vi "Create Level.vi"(8 "Error In":errorcluster, 10 "Selected Level":string, 11 "WAD Cluster IN":T1) -> (0 "Error Out":errorcluster, 2 "2D Picture":picture, 3 "WAD Cluster OUT":T1)   [LabVIEW 2017]
uses:
  WAD_MainCluster.ctl
  TextureList.ctl
  PatchList.ctl
  Lumps.ctl
  THINGSList.ctl
  <userlib>/_OpenG.lib/array/array.llb/Search 1D Array (String)__ogtk.vi
  <userlib>/_OpenG.lib/array/array.llb/Delete Elements from 1D Array (String)__ogtk.vi
  <userlib>/_OpenG.lib/array/array.llb/Filter 1D Array with Scalar (I32)__ogtk.vi
  <vilib>/picture/picture.llb/Draw 8-Bit Pixmap.vi
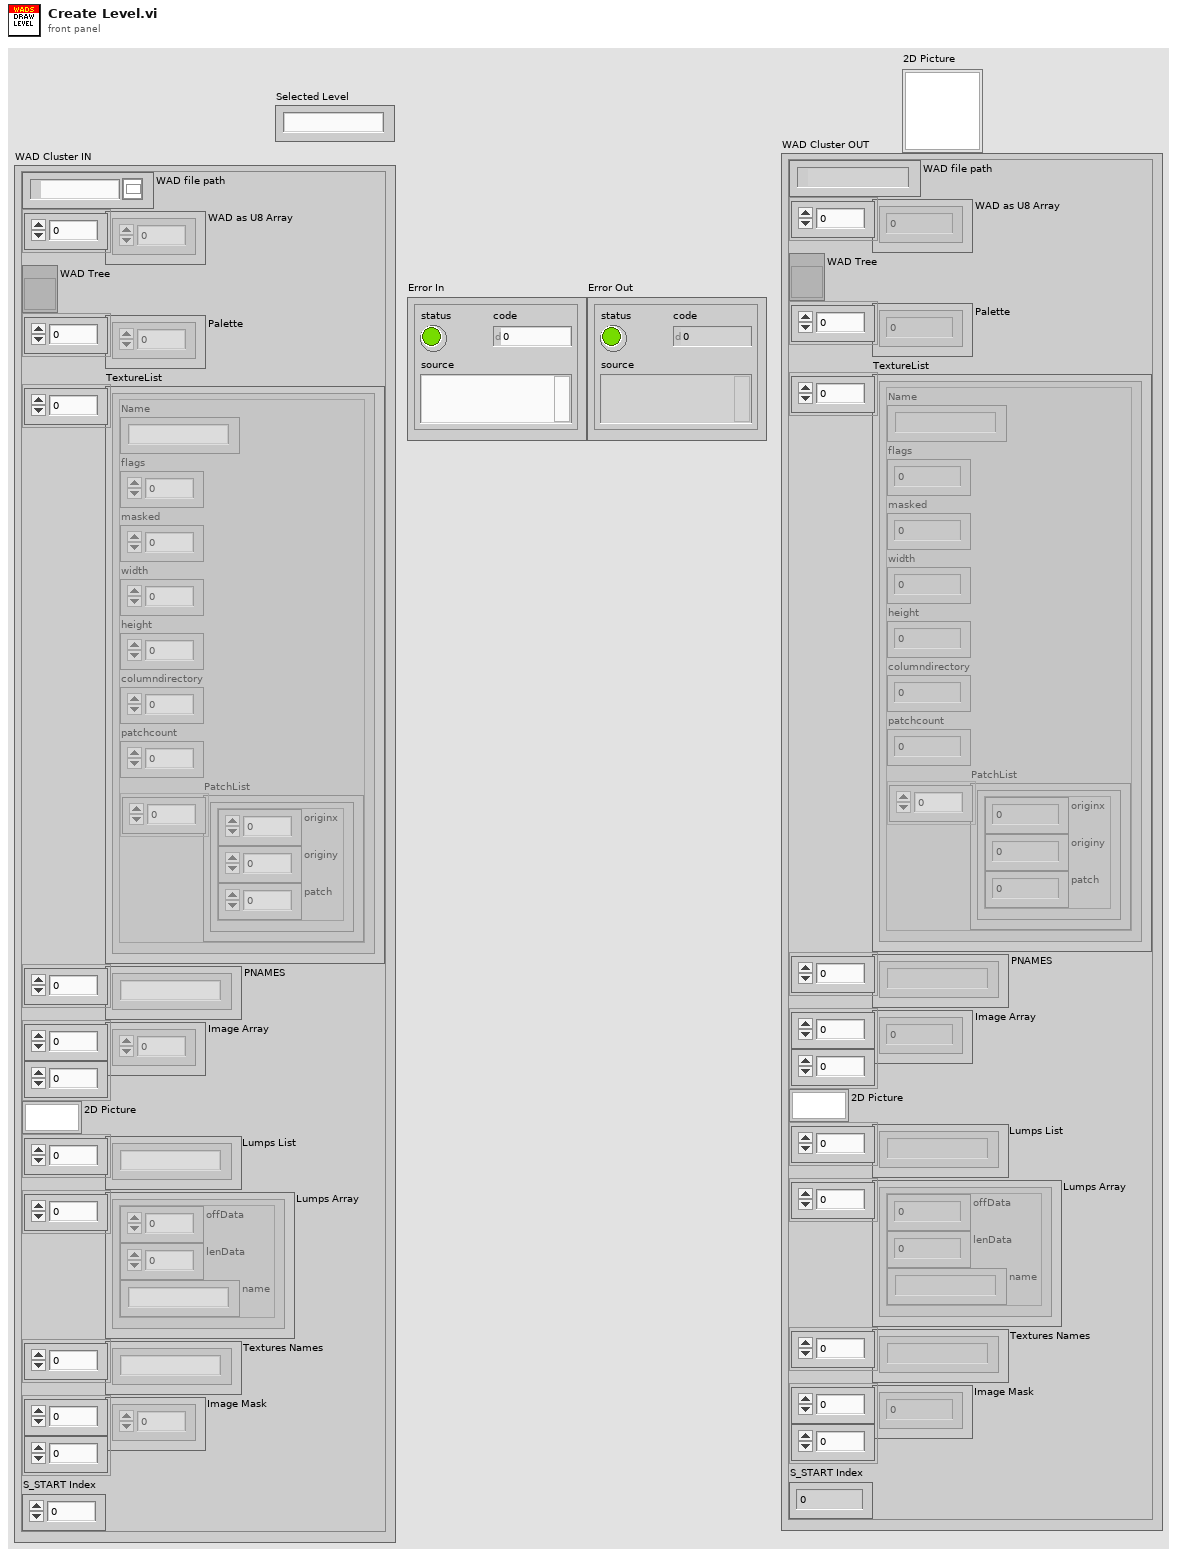
[diagram p1: front panel]
types:
  T1 = typedef "WAD_MainCluster.ctl" = cluster{"WAD file path":path, "WAD as U8 Array":u8[], "WAD Tree":refnum<vi>, "Palette":u32[], "TextureList":T2[], "PNAMES":string[], "Image Array":i16[][], "2D Picture":picture, "Lumps List":string[], "Lumps Array":T4[], "Textures Names":string[], "Image Mask":i16[][], "S_START Index":i32}
  T2 = typedef "TextureList.ctl" = cluster{"Name":string, "flags":u16, "masked":i16, "width":i16, "height":i16, "columndirectory":u32, "patchcount":i16, "PatchList":T3[]}
  T3 = typedef "PatchList.ctl" = cluster{"originx":i16, "originy":i16, "patch":i16}
  T4 = typedef "Lumps.ctl" = cluster{"offData":i32, "lenData":i32, "name":string}
  T5 = cluster{"left":i16, "top":i16, "right":i16, "bottom":i16}
  T6 = typedef "THINGSList.ctl" = string[][]
  T7 = cluster{"filtered array[0]":i32, "filtered array[1]":i32}
  T8 = typedef "PatchHeader.ctl" = cluster{"Width":u16, "Height":u16, "XOffset":i16, "YOffset":i16}
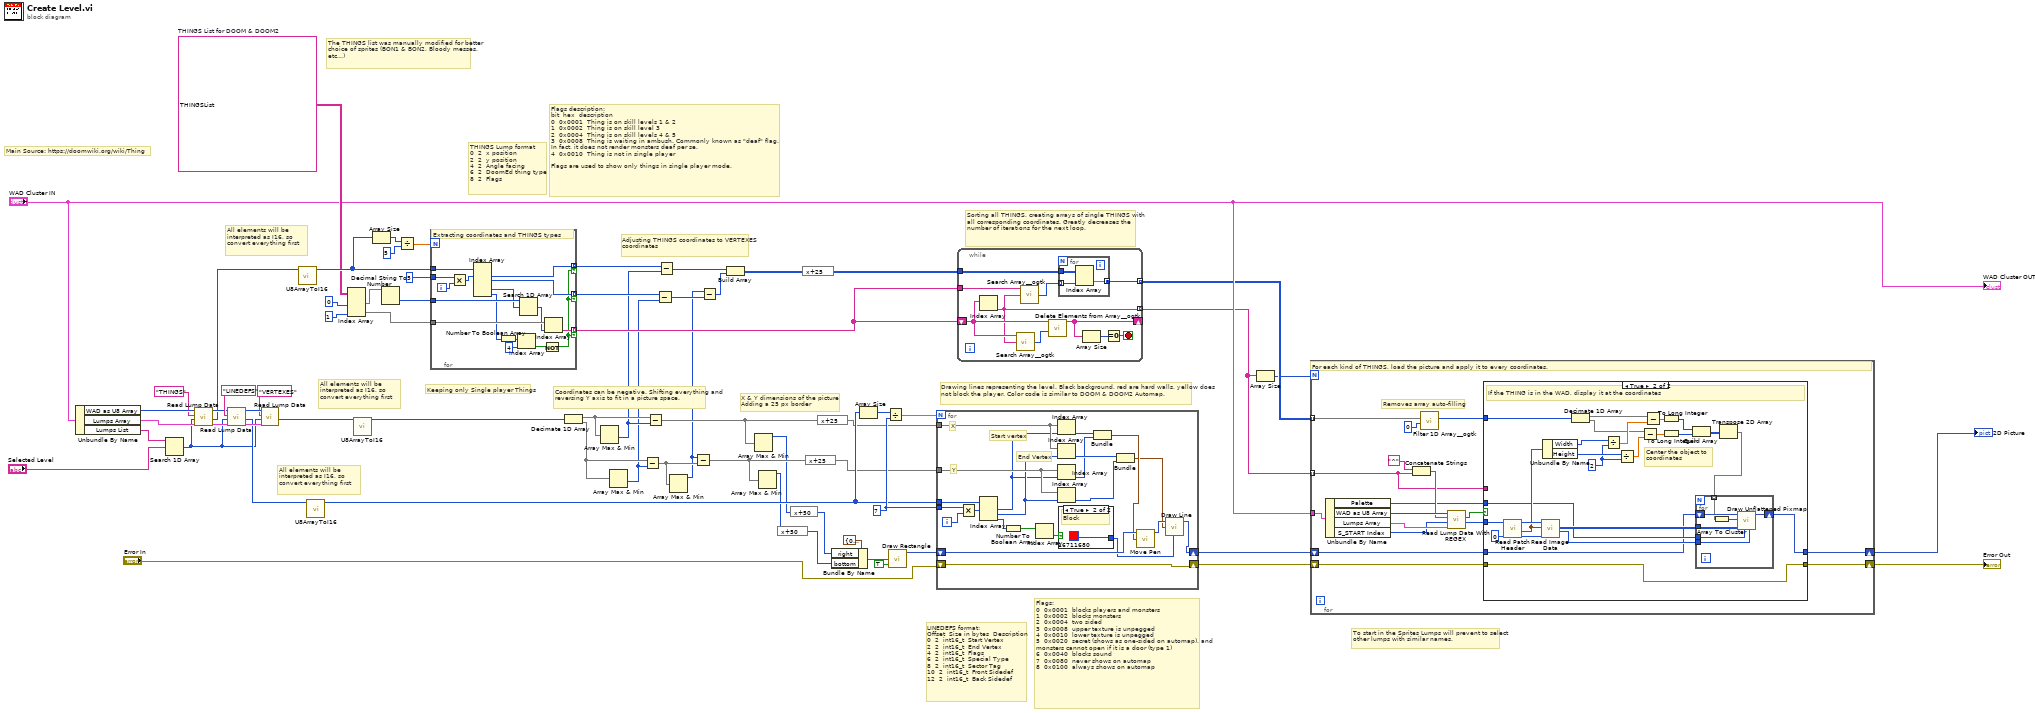
[diagram p0: block diagram]
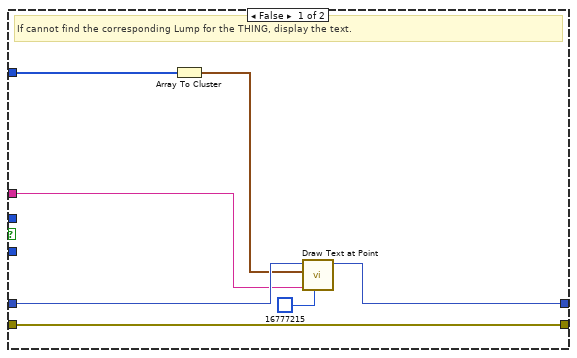
[diagram p2: hidden frame]
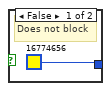
[diagram p3: hidden frame]
diagram:
  w21 = T6 [["1", "PLAY"], ["2", "PLAY"], ["3", "PLAY"], ["4", "PLAY"], ["5", "BKEY"], ["6", "YKEY"], ["7", "SPID"], ["8", "BPAK"], ["9", "SPOS"], ["10", "PLAYN"], ["11", "DM Spawn"], ["12", "PLAYW"], ["13", "RKEY"], ["14", "Teleport"], ["15", "PLAYN"], ["16", "CYBR"], ["17", "CELP"], ["18", "POSSL"], ["19", "SPOSL"], ["20", "TROOM"], ["21", "SARGN"], ["22", "HEADL"], ["23", "SKUL"], ["24", "POL5"], ["25", "POL1"], ["26", "POL6"], ["27", "POL4"], ["28", "POL2"], ["29", "POL3"], ["30", "COL1"], ["31", "COL2"], ["32", "COL3"], ["33", "COL4"], ["34", "CAND"], ["35", "CBRA"], ["36", "COL5"], ["37", "COL6"], ["38", "RSKU"], ["39", "YSKU"], ["40", "BSKU"], ["41", "CEYE"], ["42", "FSKU"], ["43", "TRE1"], ["44", "TBLU"], ["45", "TGRN"], ["46", "TRED"], ["47", "SMIT"], ["48", "ELEC"], ["49", "GOR1"], ["50", "GOR2"], ["51", "GOR3"], ["52", "GOR4"], ["53", "GOR5"], ["54", "TRE2"], ["55", "SMBT"], ["56", "SMGT"], ["57", "SMRT"], ["58", "SARG"], ["59", "GOR2"], ["60", "GOR4"], ["61", "GOR3"], ["62", "GOR5"], ["63", "GOR1"], ["64", "VILE"], ["65", "CPOS"], ["66", "SKEL"], ["67", "FATT"], ["68", "BSPI"], ["69", "BOS2A"], ["70", "FCAN"], ["71", "PAIN"], ["72", "KEEN"], ["73", "HDB1"], ["74", "HDB2"], ["75", "HDB3"], ["76", "HDB4"], ["77", "HDB5"], ["78", "HDB6"], ["79", "POB1"], ["80", "POB2"], ["81", "BRS1"], ["82", "SGN2"], ["83", "MEGA"], ["84", "SSWV"], ["85", "TLMP"], ["86", "TLP2"], ["87", "Spawn Spot"], ["88", "BBRN"], ["89", "Monster Spawn"], ["2001", "SHOT"], ["2002", "MGUN"], ["2003", "LAUN"], ["2004", "PLAS"], ["2005", "CSAW"], ["2006", "BFUG"], ["2007", "CLIP"], ["2008", "SHEL"], ["2010", "ROCK"], ["2011", "STIM"], ["2012", "MEDI"], ["2013", "SOUL"], ["2014", "BON1D"], ["2015", "BON2D"], ["2018", "ARM1"], ["2019", "ARM2"], ["2022", "PINV"], ["2023", "PSTR"], ["2024", "PINS"], ["2025", "SUIT"], ["2026", "PMAP"], ["2028", "COLU"], ["2035", "BAR"], ["2045", "PVIS"], ["2046", "BROK"], ["2047", "CELL"], ["2048", "AMMO"], ["2049", "SBOX"], ["3001", "TROO"], ["3002", "SARG"], ["3003", "BOSS"], ["3004", "POSS"], ["3005", "HEAD"], ["3006", "SKUL"]]  # THINGS List for DOOM & DOOM2
  w56 = 7 ("index")
  # "To start in the Sprites Lumps will prevent to select other lumps with similar names."
  # "The THINGS list was manually modified for better choice of sprites (BON1 & BON2, Bloody messes, etc...)"
  # "Keeping only Single player Things"
  # "Flags:\n0 \t0x0001 \tblocks players and monsters\n1 \t0x0002 \tblocks monsters\n2 \t0x0004 \ttwo sided\n3 \t0x0008 \tupper texture is unpegged\n4 \t0x0010 \tlower texture is unpegged\n5 \t0x0020 \tsecret (shows as one-sided on automap), and monsters cannot open if it is a door (type 1)\n6 \t0x0040 \tblocks sound\n7 \t0x0080 \tnever shows on automap\n8 \t0x0100 \talways shows on automap"
  # "LINEDEFS format:\nOffset \tSize in bytes \tDescription\n0 \t2 \tint16_t \tStart Vertex\n2 \t2 \tint16_t \tEnd Vertex\n4 \t2 \tint16_t \tFlags\n6 \t2 \tint16_t \tSpecial Type\n8 \t2 \tint16_t \tSector Tag\n10 \t2 \tint16_t \tFront Sidedef\n12 \t2 \tint16_t \tBack Sidedef"
  # "Flags description:\nbit \thex \tdescription\n0 \t0x0001 \tThing is on skill levels 1 & 2\n1 \t0x0002 \tThing is on skill level 3\n2 \t0x0004 \tThing is on skill levels 4 & 5\n3 \t0x0008 \tThing is waiting in ambush. Commonly known as \"deaf\" flag.\nIn fact, it does not render monsters deaf per se.\n4 \t0x0010 \tThing is not in single player \n\nFlags are used to show only things in single player mode."
  # "Coordinates can be negative. Shifting everything and reversing Y axis to fit in a picture space."
  # "X & Y dimensions of the picture\nAdding a 25 px border"
  # "Drawing lines representing the level. Black background, red are hard walls, yellow does not block the player. Color code is similar to DOOM & DOOM2 Automap."
  # "Main Source: https://doomwiki.org/wiki/Thing"
  # "All elements will be interpreted as I16, so convert everything first"
  # "All elements will be interpreted as I16, so convert everything first"
  # "All elements will be interpreted as I16, so convert everything first"
  # "THINGS Lump format\n0 \t2 \tx position\n2 \t2 \ty position\n4 \t2 \tAngle facing\n6 \t2 \tDoomEd thing type\n8 \t2 \tFlags"
  # "Sorting all THINGS, creating arrays of single THINGS with all corresponding coordinates. Greatly decreases the number of iterations for the next loop."
  # "Adjusting THINGS coordinates to VERTEXES coordinates"
  n1 = Unbundle By Name("WAD Cluster IN") -> ("WAD as U8 Array"=w65:u8[], "Lumps Array"=w64:T4[], "Lumps List"=w60:string[])
  n2 = Search 1D Array(1D array=w60, element="Selected Level") -> (index of element=w46:i32)  [unwired: 1 in]
  n3 = call "Read Lump Data.vi"("Lumps Directory IN"=w64, "start index (0)"=w46, "Lump Name"="THINGS" ("element"), "Input U8"=w65) -> ("Lumps Directory OUT"=w66:T4[], "Lump DATA OUT"=w32:u8[], "Output U8"=w62:u8[])  [unwired: 4 in, 1 out]
  n4 = call "Read Lump Data.vi"("Lumps Directory IN"=w66, "start index (0)"=w46, "Lump Name"="LINEDEFS" ("element"), "Input U8"=w62) -> ("Lumps Directory OUT"=w52:T4[], "Lump DATA OUT"=w50:u8[], "Output U8"=w51:u8[])  [unwired: 4 in, 1 out]
  n5 = call "Read Lump Data.vi"("Lumps Directory IN"=w52, "start index (0)"=w46, "Lump Name"="VERTEXES" ("element"), "Input U8"=w51) -> ("Lump DATA OUT"=w31:u8[])  [unwired: 4 in, 3 out]
  n6 = call "U8ArrayToI16.vi"("U8 DATA IN"=w32) -> ("I16 OUT"=w44:i16[])  [unwired: 10 in]
  n7 = call "U8ArrayToI16.vi"("U8 DATA IN"=w50) -> ("I16 OUT"=w49:i16[])  [unwired: 10 in]
  n8 = Index Array(array=w21, index (col) #1=0, index (col) #2=1) -> (element #1=w23:string[], element #2=w22:string[])  [unwired: 2 in]
  n9 = call "U8ArrayToI16.vi"("U8 DATA IN"=w31) -> ("I16 OUT"=w59:i16[])  [unwired: 10 in]
  n10 = Array Size(array=w44) -> (size(s)=w48:i32)
  n11 = Decimal String To Number(string=w23) -> (number=w42:i32[])  [unwired: 2 in, 1 out]
  n12 = Divide(x=w48, y=5 ("index")) -> (x/y=w45:dbl)
  n13 = for {
    N: w45 -> [_]
    tunnel: w44 -> [w81]
    tunnel: 5 ("index") -> [w80]
    tunnel: w22 -> [w78]
    tunnel: w42 -> [w76]
    tunnel: [w77] -> w41 mode=indexing if=w67
    tunnel: [w75] -> w27 mode=indexing if=w67
    tunnel: [w74] -> w29 mode=indexing if=w67
    i -> [w79]
    # "Extracting coordinates and THINGS types"
    n14 = Multiply(x=w80, y=w79) -> (x*y=w82:i32)
    n15 = Index Array(array=w81, index #1=w82) -> (element #1=w75:i16, element #2=w74:i16, element #4=w73:i16, element #5=w70:i16)  [unwired: 4 in, 1 out]
    n16 = Number To Boolean Array(number=w70) -> (Boolean array=w71:bool[])
    n17 = Index Array(array=w71, index=4) -> (element=w68:bool)
    n18 = Search 1D Array(1D array=w76, element=w73) -> (index of element=w72:i32)  [unwired: 1 in]
    n19 = Not(x=w68) -> (.not. x?=w67:bool)
    n20 = Index Array(array=w78, index=w72) -> (element=w77:string)
  }
  n21 = Decimate 1D Array(w59) -> (w55:i16[], w54:i16[])
  n22 = Array Max & Min(array=w55) -> (min value=w28:i16)  [unwired: 3 out]
  n23 = Array Max & Min(array=w54) -> (min value=w26:i16)  [unwired: 3 out]
  n24 = Subtract(x=w54, y=w26) -> (x-y=w40:i16[])
  n25 = Subtract(x=w55, y=w28) -> (x-y=w53:i16[])
  n26 = Subtract(x=w29, y=w26) -> (x-y=w38:i16[])
  n27 = Subtract(x=w27, y=w28) -> (x-y=w37:i16[])
  n28 = Array Max & Min(array=w40) -> (max value=w25:i16)  [unwired: 3 out]
  n29 = Subtract(x=w25, y=w40) -> (x-y=w39:i16[])
  n30 = Subtract(x=w25, y=w38) -> (x-y=w24:i16[])
  n31 = Build Array(w37, w24) -> (w34:i16[][])
  n32 = Array Max & Min(array=w53) -> (max value=w17:i16)  [unwired: 3 out]
  n33 = Array Max & Min(array=w39) -> (max value=w16:i16)  [unwired: 3 out]
  n34 = expression code="x+50"(w16) -> (w7:i16)
  n35 = expression code="x+50"(w17) -> (w8:i16)
  n36 = expression code="x+25"(w34) -> (w10:i16[][])
  n37 = expression code="x+25"(w39) -> (w11:i16[])
  n38 = expression code="x+25"(w53) -> (w12:i16[])
  n39 = Bundle By Name(cluster=T5 {"left"=0, "top"=0, "right"=0, "bottom"=0} ("rect"), "right"=w8, "bottom"=w7) -> (w6:T5)
  n40 = Array Size(array=w49) -> (size(s)=w58:i32)
  n41 = Divide(x=w58, y=w56) -> (x/y=w57:dbl)
  n42 = call <vilib>:"Draw Rectangle.vi"("rect"=w6, "fill?(F)"=TRUE) -> ("new picture"=w4:picture)  [unwired: 7 in]
  n43 = for {
    N: w57 -> [_]
    tunnel: w49 -> [w104]
    tunnel: w56 -> [w102]
    tunnel: w12 -> [w100]
    tunnel: w11 -> [w99]
    shift-right: [w86] -> w36
    shift-left: "Error In" -> [w86]
    shift-right: [w87] -> w14
    shift-left: w4 -> [w92]
    i -> [w103]
    # "End Vertex"
    # "Start vertex"
    # "X"
    # "Y"
    n44 = Multiply(x=w102, y=w103) -> (x*y=w101:i32)
    n45 = Index Array(array=w104, index #1=w101) -> (element #1=w97:i16, element #2=w98:i16, element #3=w96:i16)  [unwired: 2 in]
    n46 = Number To Boolean Array(number=w96) -> (Boolean array=w95:bool[])
    n47 = Index Array(array=w95) -> (element=w94:bool)  [unwired: 1 in]
    n48 = Index Array(array=w100, index=w97) -> (element=w93:i16)
    n49 = Index Array(array=w100, index=w98) -> (element=w85:i16)
    n50 = Index Array(array=w99, index=w97) -> (element=w84:i16)
    n51 = Index Array(array=w99, index=w98) -> (element=w83:i16)
    n52 = case shown="True" w94 {
      tunnel: [u32 16774656 ("Color") u32 16711680 ("Color")] -> w88
      frame False {
        # "Does not block"
      }
      frame True {
        # "Block"
      }
    }
    n53 = Bundle(w93, w84) -> (w90:cluster{i16, i16})  [unwired: 1 in]
    n54 = Bundle(w85, w83) -> (w89:cluster{i16, i16})  [unwired: 1 in]
    n55 = call <vilib>:"Move Pen.vi"("new position"=w90, "picture"=w92) -> ("new picture"=w91:picture)  [unwired: 3 in]
    n56 = call <vilib>:"Draw Line.vi"("picture"=w91, "end point"=w89, "color(black)"=w88) -> ("new picture"=w87:picture)  [unwired: 6 in]
  }
  n57 = while {
    shift-right: [w113] -> _
    shift-left: w41 -> [w116]
    tunnel: [w108] -> w15 mode=indexing
    tunnel: w10 -> [w110]
    tunnel: w41 -> [w109]
    tunnel: [w107] -> w13 mode=indexing
    stop <- w114 stop-if-true
    n58 = Index Array(array=w116) -> (element=w108:string)  [unwired: 1 in]
    n59 = call-poly <userlib>:"Search Array__ogtk.vi"("Array"=w116, "Element Data"=w108) -> ("Indices of Elements"=w112:i32[])  [unwired: 7 in]
    n60 = call-poly <userlib>:"Search Array__ogtk.vi"("Array"=w109, "Element Data"=w108) -> ("Indices of Elements"=w111:i32[])  [unwired: 7 in]
    n61 = call-poly <userlib>:"Delete Elements from Array__ogtk.vi"("indices"=w112, "array"=w116) -> ("array w/ subset deleted"=w113:string[])  [unwired: 8 in, 1 out]
    n62 = for {
      tunnel: w110 -> [w119]
      tunnel: w111 -> [w117] mode=indexing
      tunnel: [w118] -> w107 mode=concatenating
      n63 = Index Array(array=w119, index (col)=w117) -> (element=w118:i16[])  [unwired: 1 in]
    }
    n64 = Array Size(array=w113) -> (size(s)=w115:i32)
    n65 = Equal To 0?(x=w115) -> (x = 0?=w114:bool)
  }
  n66 = Array Size(array=w15) -> (size(s)=w1:i32)
  n67 = for {
    N: w1 -> [_]
    tunnel: w13 -> [w124] mode=indexing
    tunnel: w15 -> [w126] mode=indexing
    tunnel: "WAD Cluster IN" -> [w133]
    shift-right: [w131] -> w2
    shift-left: w14 -> [w122]
    shift-right: [w121] -> w35
    shift-left: w36 -> [w128]
    # "Removes array auto-filling"
    # "For each kind of THINGS, load the picture and apply it to every coordinates."
    n68 = Unbundle By Name(w133) -> ("Palette"=w127:u32[], "WAD as U8 Array"=w136:u8[], "Lumps Array"=w135:T4[], "S_START Index"=w120:i32)
    n69 = Concatenate Strings("^", w126) -> (w130:string)
    n70 = call-poly <userlib>:"Filter 1D Array__ogtk.vi"("items to filter"=u32 0 ("Index"), "array"=w124) -> ("filtered array"=w123:i32[])  [unwired: 4 in, 1 out]
    n71 = call "Read Lump Data With REGEX.vi"("Lumps Directory IN"=w135, "start index (0)"=w120, "Lump Name"=w130, "Input U8"=w136) -> ("Lump DATA OUT"=w132:u8[], "Found?"=w129:bool)  [unwired: 4 in, 2 out]
    n72 = case shown="True" w129 {
      tunnel: w123 -> [w142 w151]
      tunnel: w132 -> [_ w165]
      tunnel: [w138 w146] -> w131
      tunnel: w122 -> [w143 w147]
      tunnel: w127 -> [_ w148]
      tunnel: w128 -> [w139 w145]
      tunnel: [w139 w145] -> w121
      tunnel: w126 -> [w140 _]
      frame False {
        # "If cannot find the corresponding Lump for the THING, display the text."
        n73 = Array To Cluster(array=w142) -> (cluster=w141:T7)
        n74 = call <vilib>:"Draw Text at Point.vi"("text color(black)"=u32 16777215, "text"=w140, "origin"=w141, "picture"=w143) -> ("new picture"=w138:picture)  [unwired: 6 in, 1 out]
      }
      frame True {
        w155 = u32 2 ("Index")
        # "Center the object to coordinates"
        # "If the THING is in the WAD, display it at the coordinates"
        n75 = call "Read Patch Header.vi"("Index"=u32 0, "Patch DATA IN"=w165) -> ("Index+8"=w167:u32, "PatchHeader"=w164:T8, "Patch DATA OUT"=w168:u8[])  [unwired: 7 in]
        n76 = call "Read Image Data.vi"("Input Index"=w167, "PatchHeader"=w164, "Patch DATA IN"=w168) -> ("Mask OUT"=w149:u8[], "Image OUT"=w150:u8[][])  [unwired: 5 in, 2 out]
        n77 = Unbundle By Name(w164) -> ("Width"=w163:u16, "Height"=w156:u16)
        n78 = Decimate 1D Array(w151) -> (w162:i32[], w153:i32[])
        n79 = Divide(x=w163, y=w155) -> (x/y=w160:dbl)
        n80 = Divide(x=w156, y=w155) -> (x/y=w154:dbl)
        n81 = Subtract(x=w153, y=w154) -> (x-y=w152:dbl[])
        n82 = Subtract(x=w162, y=w160) -> (x-y=w161:dbl[])
        n83 = To Long Integer(number=w161) -> (32bit integer=w159:i32[])
        n84 = To Long Integer(number=w152) -> (32bit integer=w158:i32[])
        n85 = Build Array(w159, w158) -> (w157:i32[][])
        n86 = Transpose 2D Array(2D array=w157) -> (transposed array=w144:i32[][])
        n87 = for {
          tunnel: w150 -> [w175]
          tunnel: w149 -> [w174]
          tunnel: w148 -> [w173]
          shift-right: [w171] -> w146
          shift-left: w147 -> [w172]
          tunnel: w144 -> [w170] mode=indexing
          n88 = Array To Cluster(array=w170) -> (cluster=w169:cluster{"[0]":i32, "[1]":i32})
          n89 = call-poly <vilib>:"Draw Unflattened Pixmap.vi"("picture"=w172, "top left point(0, 0)"=w169, "data"=w175, "color table"=w173, "mask"=w174) -> ("new picture"=w171:picture)  [unwired: 4 in]
        }
      }
    }
  }
  "Error Out" <- w35
  "2D Picture" <- w2
  "WAD Cluster OUT" <- "WAD Cluster IN"
